vi "Error Handler.vi"(8 "error in (no error)":errorcluster caption="Error IN", 9 "error code":i32 caption="ErrorCode", 10 "language":u32=1, 11 "deviceHandle":i32) -> (0 "error out":errorcluster caption="Error OUT", 3 "deviceHandle Out":i32)   [LabVIEW 2016]
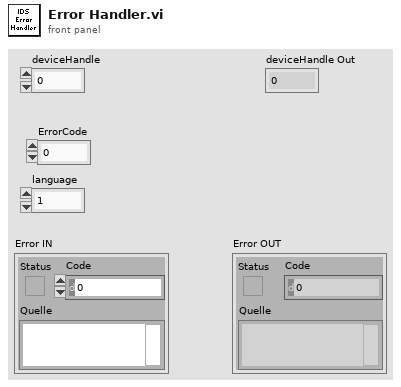
[diagram p1: front panel]
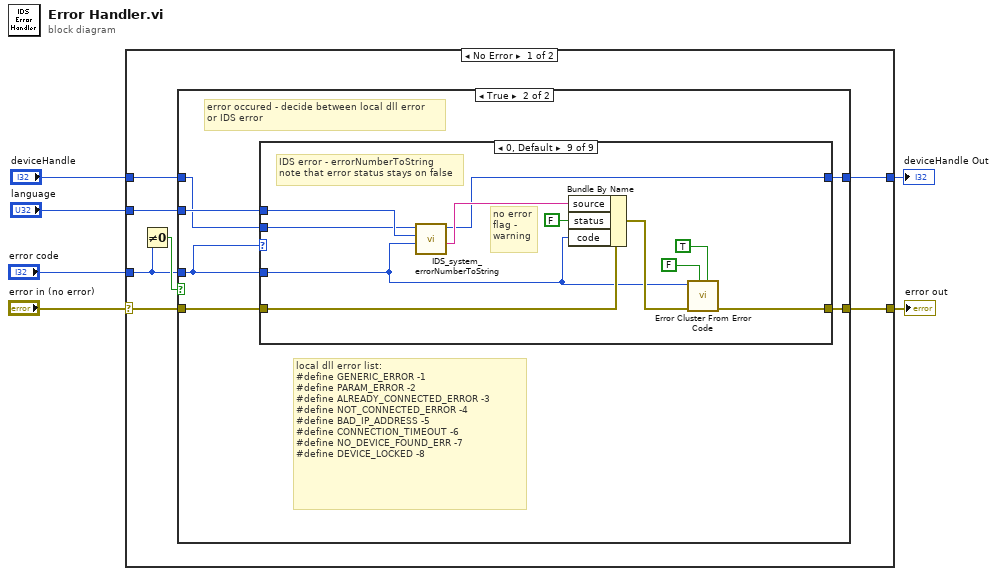
[diagram p0: block diagram]
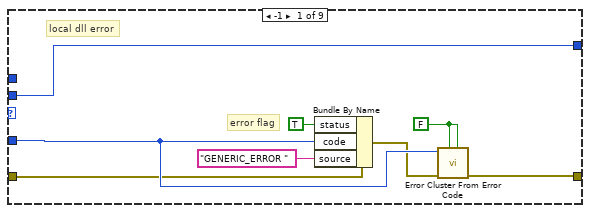
[diagram p3: hidden frame]
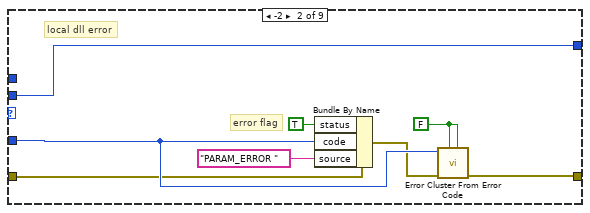
[diagram p4: hidden frame]
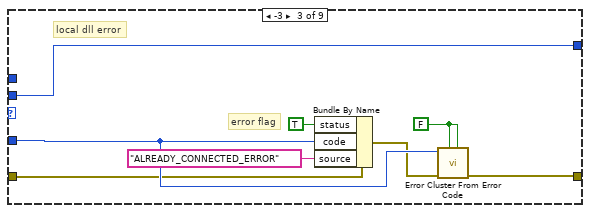
[diagram p5: hidden frame]
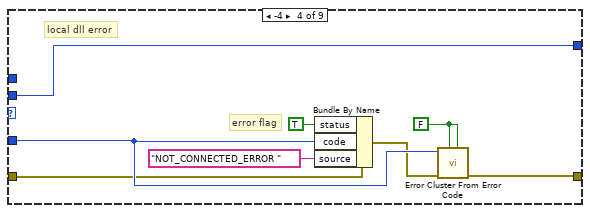
[diagram p6: hidden frame]
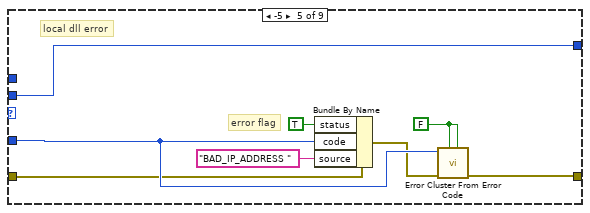
[diagram p7: hidden frame]
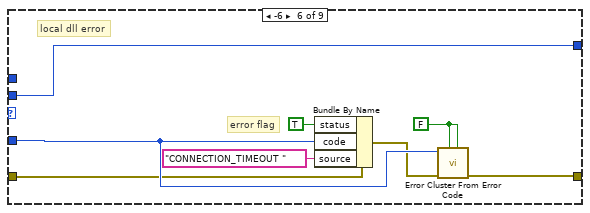
[diagram p8: hidden frame]
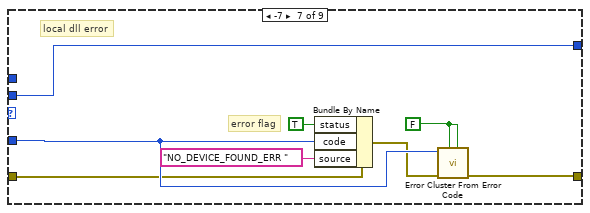
[diagram p9: hidden frame]
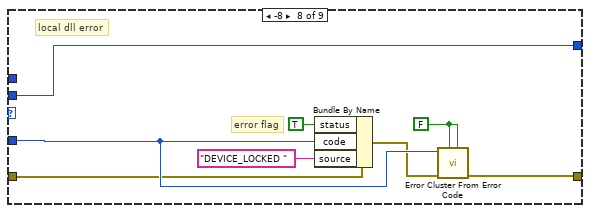
[diagram p10: hidden frame]
diagram:
  n1 = case shown="No Error" "error in (no error)" {
    selector: "error in (no error)" -> [w12 w98]
    tunnel: [w10 w98] -> w5
    tunnel: "error code" -> [w11 _]
    tunnel: "language" -> [w9 _]
    tunnel: "deviceHandle" -> [w8 w97]
    tunnel: [w7 w97] -> w1
    frame No Error {
      n2 = Not Equal To 0?(x=w11) -> (x != 0?=w13:bool)
      n3 = case shown="True" w13 {
        tunnel: w12 -> [w15 w20]
        tunnel: w11 -> [_ w16]
        tunnel: [w15 w21] -> w10
        tunnel: w9 -> [_ w19]
        tunnel: w8 -> [w14 w18]
        tunnel: [w14 w17] -> w7
        frame False {
          # "no error occured"
        }
        frame True {
          # "local dll error list:\n#define GENERIC_ERROR -1\n#define PARAM_ERROR -2\n#define ALREADY_CONNECTED_ERROR -3\n#define NOT_CONNECTED_ERROR -4\n#define BAD_IP_ADDRESS -5\n#define CONNECTION_TIMEOUT -6\n#define NO_DEVICE_FOUND_ERR -7\n#define DEVICE_LOCKED -8"
          # "error occured - decide between local dll error\nor IDS error"
          n4 = case shown="0, Default" w16 {
            tunnel: [w25 w33 w41 w49 w57 w65 w73 w82 w96] -> w21
            tunnel: w20 -> [w24 w32 w40 w48 w56 w64 w72 w81 w94]
            tunnel: w19 -> [_ _ _ _ _ _ _ _ w91]
            tunnel: w16 -> [w27 w35 w43 w51 w59 w67 w75 w84 w89]
            tunnel: w18 -> [w23 w31 w39 w47 w55 w63 w71 w80 w88]
            tunnel: [w23 w31 w39 w47 w55 w63 w71 w80 w87] -> w17
            frame -1 {
              w22 = FALSE ("show call chain? (False)")
              # "error flag"
              # "local dll error"
              n5 = Bundle By Name(cluster=w24, "status"=TRUE, "code"=w27, "source"="GENERIC_ERROR ") -> (w26:errorcluster)
              n6 = call <vilib>:"Error Cluster From Error Code.vi"("is warning? (False)"=w22, "show call chain? (False)"=w22, "error in (no error)"=w26, "error code (0)"=w27) -> ("error out"=w25:errorcluster)  [unwired: 5 in]
            }
            frame -2 {
              w30 = FALSE ("show call chain? (False)")
              # "error flag"
              # "local dll error"
              n7 = Bundle By Name(cluster=w32, "status"=TRUE, "code"=w35, "source"="PARAM_ERROR ") -> (w34:errorcluster)
              n8 = call <vilib>:"Error Cluster From Error Code.vi"("is warning? (False)"=w30, "show call chain? (False)"=w30, "error in (no error)"=w34, "error code (0)"=w35) -> ("error out"=w33:errorcluster)  [unwired: 5 in]
            }
            frame -3 {
              w38 = FALSE ("show call chain? (False)")
              # "error flag"
              # "local dll error"
              n9 = Bundle By Name(cluster=w40, "status"=TRUE, "code"=w43, "source"="ALREADY_CONNECTED_ERROR") -> (w42:errorcluster)
              n10 = call <vilib>:"Error Cluster From Error Code.vi"("is warning? (False)"=w38, "show call chain? (False)"=w38, "error in (no error)"=w42, "error code (0)"=w43) -> ("error out"=w41:errorcluster)  [unwired: 5 in]
            }
            frame -4 {
              w46 = FALSE ("show call chain? (False)")
              # "error flag"
              # "local dll error"
              n11 = Bundle By Name(cluster=w48, "status"=TRUE, "code"=w51, "source"="NOT_CONNECTED_ERROR ") -> (w50:errorcluster)
              n12 = call <vilib>:"Error Cluster From Error Code.vi"("is warning? (False)"=w46, "show call chain? (False)"=w46, "error in (no error)"=w50, "error code (0)"=w51) -> ("error out"=w49:errorcluster)  [unwired: 5 in]
            }
            frame -5 {
              w54 = FALSE ("show call chain? (False)")
              # "error flag"
              # "local dll error"
              n13 = Bundle By Name(cluster=w56, "status"=TRUE, "code"=w59, "source"="BAD_IP_ADDRESS ") -> (w58:errorcluster)
              n14 = call <vilib>:"Error Cluster From Error Code.vi"("is warning? (False)"=w54, "show call chain? (False)"=w54, "error in (no error)"=w58, "error code (0)"=w59) -> ("error out"=w57:errorcluster)  [unwired: 5 in]
            }
            frame -6 {
              w62 = FALSE ("show call chain? (False)")
              # "error flag"
              # "local dll error"
              n15 = Bundle By Name(cluster=w64, "status"=TRUE, "code"=w67, "source"="CONNECTION_TIMEOUT ") -> (w66:errorcluster)
              n16 = call <vilib>:"Error Cluster From Error Code.vi"("is warning? (False)"=w62, "show call chain? (False)"=w62, "error in (no error)"=w66, "error code (0)"=w67) -> ("error out"=w65:errorcluster)  [unwired: 5 in]
            }
            frame -7 {
              w70 = FALSE ("show call chain? (False)")
              # "error flag"
              # "local dll error"
              n17 = Bundle By Name(cluster=w72, "status"=TRUE, "code"=w75, "source"="NO_DEVICE_FOUND_ERR ") -> (w74:errorcluster)
              n18 = call <vilib>:"Error Cluster From Error Code.vi"("is warning? (False)"=w70, "show call chain? (False)"=w70, "error in (no error)"=w74, "error code (0)"=w75) -> ("error out"=w73:errorcluster)  [unwired: 5 in]
            }
            frame -8 {
              w78 = FALSE ("show call chain? (False)")
              # "error flag"
              # "local dll error"
              n19 = Bundle By Name(cluster=w81, "status"=TRUE, "code"=w84, "source"="DEVICE_LOCKED ") -> (w83:errorcluster)
              n20 = call <vilib>:"Error Cluster From Error Code.vi"("is warning? (False)"=w78, "show call chain? (False)"=w78, "error in (no error)"=w83, "error code (0)"=w84) -> ("error out"=w82:errorcluster)  [unwired: 5 in]
            }
            frame 0, Default {
              # "no error\nflag - \nwarning"
              # "IDS error - errorNumberToString\nnote that error status stays on false"
              n21 = call "IDS_system_errorNumberToString.vi"("errorNumber"=w89, "language"=w91, "deviceHandle"=w88) -> ("error String"=w90:string, "deviceHandle out"=w87:i32)  [unwired: 7 in]
              n22 = Bundle By Name(cluster=w94, "source"=w90, "status"=FALSE, "code"=w89) -> (w92:errorcluster)
              n23 = call <vilib>:"Error Cluster From Error Code.vi"("is warning? (False)"=TRUE, "show call chain? (False)"=FALSE, "error in (no error)"=w92, "error code (0)"=w89) -> ("error out"=w96:errorcluster)  [unwired: 5 in]
            }
          }
        }
      }
    }
    frame Error {
    }
  }
  "error out" <- w5
  "deviceHandle Out" <- w1
